vi "Rotated Holder.vi"(8 "error in (no error)":errorcluster, 11 "Box Length Y 3":sgl) -> (0 "error out":errorcluster, 3 "SceneObject out":refnum<vi>)   [LabVIEW 2026, in "XRay CArm.lvclass"]
uses:
  XRay CArm.lvclass
  <vilib>/picture/3D Picture Control/Object/Create Object (drawable).vi
  <vilib>/picture/3D Picture Control/Object/Add Object (reference).vi
  <vilib>/picture/3D Picture Control/NI_3D Picture Control.lvlib
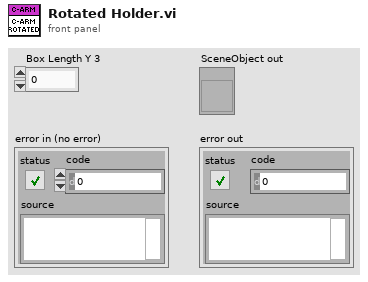
[diagram p1: front panel]
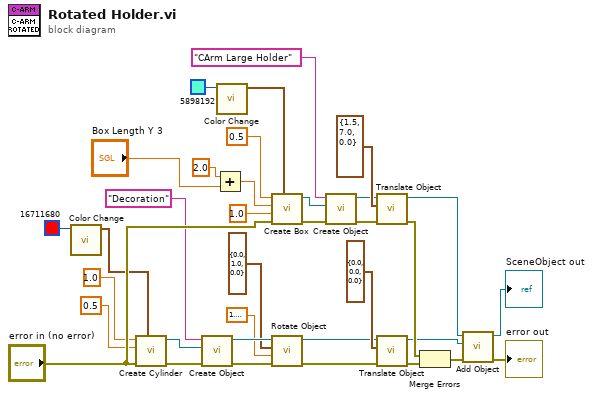
[diagram p0: block diagram]
diagram:
  n1 = call <vilib>:"Color Change.vi"("Color"=u32 16711680) -> ("RGBA"=w21:cluster{"R":sgl, "G":sgl, "B":sgl, "A":sgl})  [unwired: 10 in]
  n2 = call <vilib>:"Create Cylinder.vi"("Color"=w21, "error in (no error)"="error in (no error)", "Radius"=sgl 0.5, "Height"=sgl 1.0) -> ("error out"=w15:errorcluster, "New Cylinder Refnum"=w16:refnum<vi>)  [unwired: 6 in]
  n3 = call-poly <vilib>:"Create Object.vi"("error in (no error)"=w15, "Geometry"=w16, "Name"="Decoration") -> ("error out"=w27:errorcluster, "Scene:New Object"=w14:refnum<vi>)  [unwired: 7 in]
  n4 = Add(x=sgl 2.0, y="Box Length Y 3") -> (x+y=w29:sgl)
  n5 = call <vilib>:"Color Change.vi"("Color"=u32 5898192) -> ("RGBA"=w7:cluster{"R":sgl, "G":sgl, "B":sgl, "A":sgl})  [unwired: 10 in]
  n6 = call <vilib>:"Create Box.vi"("Color"=w7, "error in (no error)"="error in (no error)", "Length Z"=sgl 1.0 ("Box Length Z 3"), "Length Y"=w29, "Length X"=sgl 0.5 ("Box Length X 3")) -> ("error out"=w5:errorcluster, "New Box Refnum"=w4:refnum<vi>)  [unwired: 5 in]
  n7 = call <vilib>:"Rotate Object.vi"("error in (no error)"=w27, "Angle"=1.5707963267948966, "Axis"=cluster{"X":sgl, "Y":sgl, "Z":sgl} {"X"=0.0, "Y"=1.0, "Z"=0.0}, "Scene.Object In"=w14) -> ("error out"=w28:errorcluster, "Scene.Object Out"=w13:refnum<vi>)  [unwired: 6 in]
  n8 = call-poly <vilib>:"Create Object.vi"("error in (no error)"=w5, "Geometry"=w4, "Name"="CArm Large Holder") -> ("error out"=w25:errorcluster, "Scene:New Object"=w9:refnum<vi>)  [unwired: 7 in]
  n9 = call <vilib>:"Translate Object.vi"("error in (no error)"=w25, "Translation"=cluster{"X":sgl, "Y":sgl, "Z":sgl} {"X"=1.5, "Y"=7.0, "Z"=0.0} ("Translation 2"), "Scene.Object In"=w9) -> ("error out"=w32:errorcluster, "Scene.Object Out"=w24:refnum<vi>)  [unwired: 7 in]
  n10 = call <vilib>:"Translate Object.vi"("error in (no error)"=w28, "Translation"=cluster{"X":sgl, "Y":sgl, "Z":sgl} {"X"=0.0, "Y"=0.0, "Z"=0.0} ("Translation 4"), "Scene.Object In"=w13) -> ("error out"=w33:errorcluster, "Scene.Object Out"=w26:refnum<vi>)  [unwired: 7 in]
  n11 = Merge Errors(w32, w33) -> (w34:errorcluster)
  n12 = call-poly <vilib>:"Add Object.vi"("error in (no error)"=w34, "New Object In"=w26, "Scene Object In"=w24) -> ("error out"=→"error out":errorcluster, "Scene Object Out"=→"SceneObject out":refnum<vi>)  [unwired: 6 in, 1 out]
